vi "Get System Status.vi"(8 "error in":errorcluster, 11 "System Session":refnum<k21>) -> (0 "error out":errorcluster, 2 "output cluster":T1, 3 "System Session out":refnum<k21>)   [LabVIEW 2021, in "RT Main.lvlib"]
uses:
  RT Main.lvlib
  Libraries/Common RT/Hardware Monitoring.ctl
  <resource>/objmgr/nisysapi.rc
  <resource>/objmgr/nicontrollersysapi.rc
  Libraries/Common RT/Common RT.lvlib
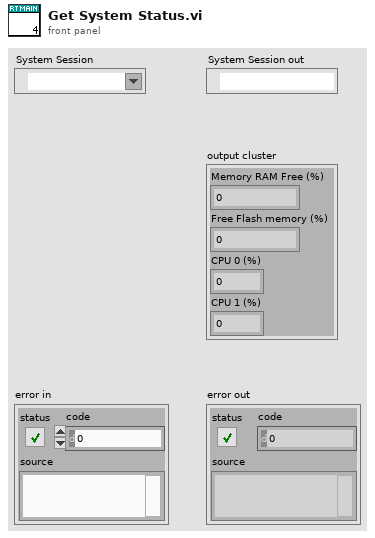
[diagram p1: front panel]
types:
  T1 = typedef "Common RT.lvlib/Hardware Monitoring.ctl" = cluster{"Memory RAM Free (%)":dbl, "Free Flash memory (%)":dbl, "CPU 0 (%)":u32, "CPU 1 (%)":u32}
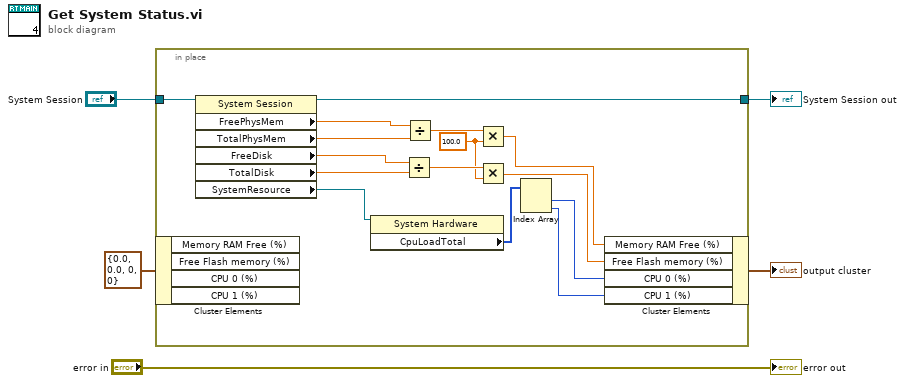
[diagram p0: block diagram]
diagram:
  n1 = in-place {
    in-place-border: "System Session" -> [w11]
    in-place-border: [w10] -> w4
    w13 = 100.0 ("y")
    n2 = in-place-cluster #1(T1 {"Memory RAM Free (%)"=0.0, "Free Flash memory (%)"=0.0, "CPU 0 (%)"=0, "CPU 1 (%)"=0} ("element")) -> ()  [unwired: 4 out]
    n3 = property class="System Session"(reference=w11) -> (reference out=w10:refnum<k21>, "FreePhysMem"=w19:dbl, "TotalPhysMem"=w20:dbl, "FreeDisk"=w16:dbl, "TotalDisk"=w15:dbl, "SystemResource"=w17:refnum<k20>)  [unwired: 1 in, 1 out]
    n4 = property class="System Hardware"(reference=w17) -> ("CpuLoadTotal"=w12:u32[])  [unwired: 1 in, 2 out]
    n5 = Divide(x=w16, y=w15) -> (x/y=w14:dbl)
    n6 = Divide(x=w19, y=w20) -> (x/y=w18:dbl)
    n7 = Multiply(x=w18, y=w13) -> (x*y=w9:dbl)
    n8 = Multiply(x=w14, y=w13) -> (x*y=w8:dbl)
    n9 = Index Array(array=w12) -> (element #1=w7:u32, element #2=w6:u32)  [unwired: 2 in]
    n10 = in-place-cluster #1("Memory RAM Free (%)"=w9, "Free Flash memory (%)"=w8, "CPU 0 (%)"=w7, "CPU 1 (%)"=w6) -> (→"output cluster":T1)
  }
  "System Session out" <- w4
  "error out" <- "error in"
